vi "Actor Core.vi"(8 "error in (no error)":errorcluster, 11 "Menu object array in":refnum<class "Menu object array.lvclass">) -> (0 "error out":errorcluster, 3 "Actor Framework.lvlib:Actor":refnum<class "Actor.lvclass">)   [LabVIEW 2015, in "Menu object array.lvclass"]
uses:
  Menu object array.lvclass
  <vilib>/ActorFramework/Actor/Actor.lvclass
  Controls/Menu object array.ctl
  Controls/Menu object.ctl
  Menu object array.lvclass/Menu object array.ctl
  <vilib>/ActorFramework/Actor/Actor.lvclass/Actor.ctl
  <vilib>/ActorFramework/Message Enqueuer/Message Enqueuer.lvclass/Message Enqueuer.ctl
  Mag Lab Measure Interface Messages/Open menu object parameters Msg/Open menu object parameters Msg.lvclass/Open menu object parameters Msg.ctl
  <vilib>/ActorFramework/Message Enqueuer/Init from Existing Queue.vi
  <vilib>/ActorFramework/Message Enqueuer/Enqueue.vi
  <vilib>/ActorFramework/Message Priority Queue/Priority Enqueue.vi
  <vilib>/ActorFramework/Message Enqueuer/Message Enqueuer.lvclass
  <vilib>/ActorFramework/Stop Msg/Stop Msg.lvclass
  Mag Lab Measure Interface Messages/Open menu object parameters Msg/Open menu object parameters Msg.lvclass
  Mag Lab Measure Interface/Mag Lab Measure UI.lvclass
panel:
  in  "test":bool
  in  "Menu object array":T1 {"Object name" items=["Select one"]}
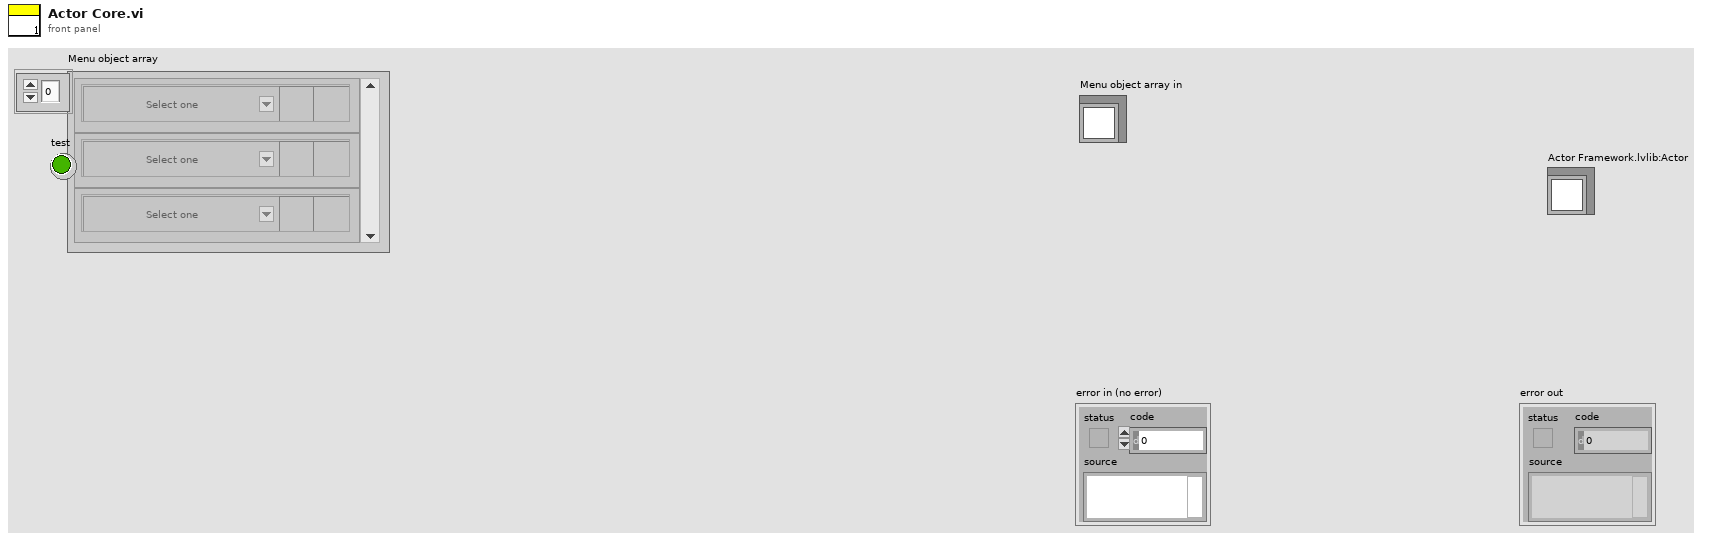
[diagram p1: front panel]
types:
  T1 = typedef "Menu object array.ctl" = T2[]
  T2 = typedef "Menu object.ctl" = cluster{"Object name":u16, "Open parameters":bool, "Remove Button":bool}
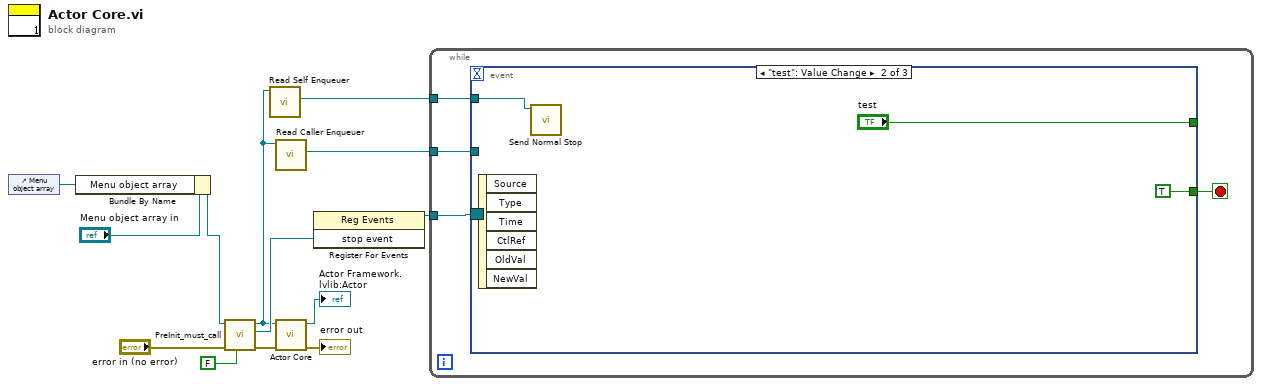
[diagram p0: block diagram]
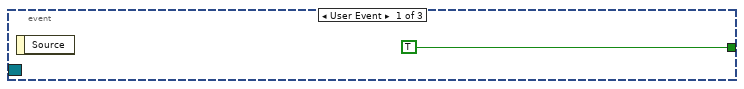
[diagram p2: hidden frame]
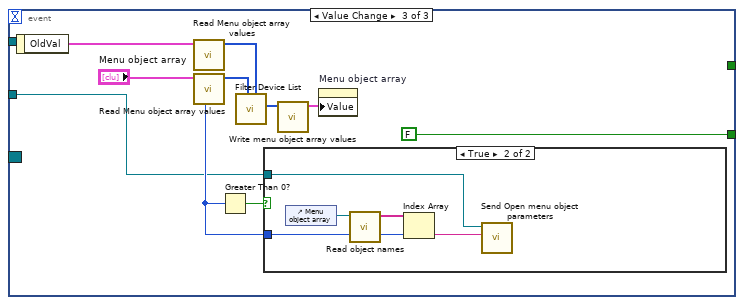
[diagram p3: hidden frame]
diagram:
  n1 = control-ref of="Menu object array"() -> (w4:refnum<vi>)
  n2 = Bundle By Name(cluster="Menu object array in", "Menu object array"=w4) -> (w5:refnum<class "Menu object array.lvclass">)
  n3 = call-dynamic "PreInit_must_call.vi"("Open Actor Core front panel? (T)"=FALSE, "error in (no error)"="error in (no error)", "Mag Lab Measure Interface in"=w5) -> ("error out"=w11:errorcluster, "stop event"=w7:refnum<user-event>, "Mag Lab Measure Interface out"=w2:refnum<class "Menu object array.lvclass">)  [unwired: 6 in]
  n4 = call <vilib>:"Read Self Enqueuer.vi"("Actor"=w2) -> ("Self Enqueuer"=w1:refnum<class "Message Enqueuer.lvclass">)  [unwired: 10 in]
  n5 = call <vilib>:"Read Caller Enqueuer.vi"("Actor"=w2) -> ("Caller Enqueuer"=w8:refnum<class "Message Enqueuer.lvclass">)  [unwired: 10 in]
  n6 = call-parent "Actor Core.vi"("error in (no error)"=w11, "Mag Lab Measure Interface in"=w2) -> ("error out"=→"error out":errorcluster, "Actor Framework.lvlib:Actor"=→"Actor Framework.lvlib:Actor":refnum<class "Actor.lvclass">)  [unwired: 8 in]
  n7 = register-events(w7) -> (reference out=w6:refnum<event-registration>)  [unwired: 2 in, 1 out]
  n8 = while {
    tunnel: w6 -> [w16]
    tunnel: w8 -> [w15]
    tunnel: w1 -> [w14]
    stop <- w17 stop-if-true
    n9 = event shown="[1] \"test\": Value Change" {
      selector: w16 -> [_ _ _]
      dyn-events: _ -> [_ _ _]
      timeout: _ -> [_ _ _]
      tunnel: [TRUE TRUE FALSE] -> w17
      tunnel: w15 -> [_ _ w22]
      tunnel: w14 -> [_ w21 _]
      tunnel: [_ "test" _] -> _
      event User Event {
        n10 = event-data() -> ()  [unwired: 1 in, 1 out]
      }
      event "test": Value Change {
        n11 = event-data() -> ()  [unwired: 1 in, 6 out]
        n12 = call <vilib>:"Send Normal Stop.vi"("Message Enqueuer"=w21) -> ()  [unwired: 10 in, 1 out]
      }
      event Value Change {
        n13 = event-data() -> ("OldVal"=w30:T1)  [unwired: 1 in]
        n14 = call "Read Menu object array values.vi"("Menu object array"=w30) -> ("Values"=w28:u16[])  [unwired: 6 in, 4 out]
        n15 = call "Read Menu object array values.vi"("Menu object array"="Menu object array") -> ("Values"=w29:u16[], "Open parameters for object"=w23:i32)  [unwired: 6 in, 3 out]
        n16 = Greater Than 0?(x=w23) -> (x > 0?=w24:bool)
        n17 = call "Filter Device List.vi"("Old List"=w28, "New List"=w29) -> ("Filtered List"=w26:u16[])  [unwired: 9 in]
        n18 = case shown="True" w24 {
          tunnel: w23 -> [_ w34]
          tunnel: w22 -> [_ w33]
          frame False {
          }
          frame True {
            n19 = control-ref of="Menu object array"() -> (w36:refnum<vi>)
            n20 = call "Read object names.vi"("Menu object array ref"=w36) -> ("Object names"=w35:string[])  [unwired: 9 in, 1 out]
            n21 = Index Array(array=w35, index=w34) -> (element=w32:string)
            n22 = call "Send Open menu object parameters.vi"("Object name"=w32, "Message Enqueuer"=w33) -> ()  [unwired: 8 in, 2 out]
          }
        }
        n23 = call "Write menu object array values.vi"("Values"=w26) -> ("Menu object array"=w25:T1)  [unwired: 10 in]
        n24 = property on="Menu object array" class="Arr"("Value"=w25) -> ()  [unwired: 2 in, 2 out]
      }
    }
  }
